vi "CC Greyout Table Row.vi"(7 "Color Box":u32(colorbox), 8 "error in (no error)":errorcluster, 9 "Color":enum16{"White", "Gray", "Custom"}(ring), 10 "Row":i32, 11 "Queue ref":refnum<vi>) -> (0 "error out":errorcluster)   [LabVIEW 2024]
uses:
  <vilib>/Utility/miscctls.llb/LVRowAndColumnTypeDef.ctl
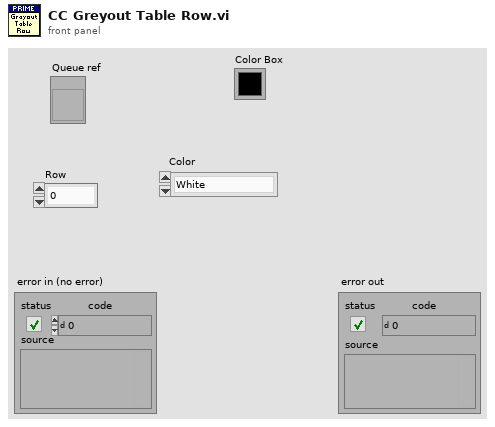
[diagram p1: front panel]
types:
  T1 = typedef "LVRowAndColumnTypeDef.ctl" = cluster{"Row":i32, "Column":i32}
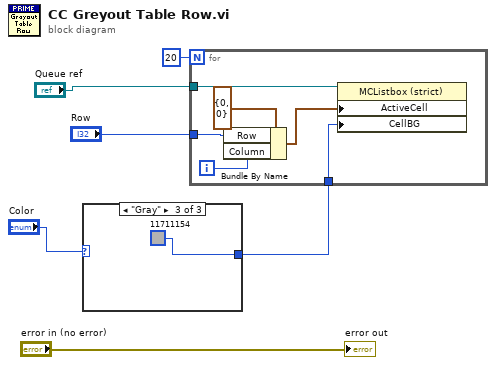
[diagram p0: block diagram]
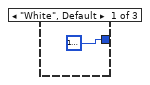
[diagram p2: hidden frame]
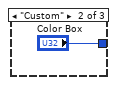
[diagram p3: hidden frame]
diagram:
  n1 = case shown="\"Gray\"" "Color" {
    tunnel: [u32 16777233 ("Color Box 2") "Color Box" u32 11711154 ("Color Box 2")] -> w3
    frame "White", Default {
    }
    frame "Custom" {
    }
    frame "Gray" {
    }
  }
  n2 = for {
    N: 20 -> [_]
    tunnel: "Queue ref" -> [w15]
    tunnel: "Row" -> [w13]
    tunnel: w3 -> [w10]
    i -> [w12]
    n3 = Bundle By Name(cluster=T1 {"Row"=0, "Column"=0} ("Active Cell:Active Cell"), "Row"=w13, "Column"=w12) -> (w11:T1)
    n4 = property class="MCListbox (strict)"(reference=w15, "ActiveCell"=w11, "CellBG"=w10) -> ()  [unwired: 1 in, 2 out]
  }
  "error out" <- "error in (no error)"
